vi "Load External Sources.vi"(8 "error in (no error)":errorcluster, 10 "JSON":string, 11 "BluelinesRedlines in":refnum<class "BluelinesRedlines.lvclass">) -> (0 "error out":errorcluster, 3 "BluelinesRedlines out":refnum<class "BluelinesRedlines.lvclass">)   [LabVIEW 2020, in "VolatusGUIElements.lvlib" / "BluelinesRedlines.lvclass"]
uses:
  BluelinesRedlines.lvclass
  BluelinesRedlines.lvclass/BluelinesRedlines.ctl
  <vilib>/JDP Science/JSONtext/Next JSON Value.vi
  <vilib>/JDP Science/JSONtext/String Subset.vi
  <vilib>/JDP Science/JSONtext/Parsing/Advance past next JSON Value (inlined COPY).vi
  <vilib>/JDP Science/JSONtext/Parsing/Advance past whitespace.vi
  <vilib>/JDP Science/JSONtext/Parsing/Advance past String.vi
  <vilib>/JDP Science/JSONtext/Parsing/Advance past Number.vi
  <vilib>/JDP Science/JSONtext/Parsing/Advance past Line Ending.vi
  <vilib>/JDP Science/JSONtext/Parsing/Parse Full Path or Item Name.vi
  <vilib>/JDP Science/JSONtext/Parsing/Advance past Array.vi
  <vilib>/JDP Science/JSONtext/Parsing/Advance past Object.vi
  <vilib>/JDP Science/JSONtext/support/Error Cluster From Code.vi
  <vilib>/JDP Science/JSONtext/Offset/Find Item Locations by Path.vi
  VolatusGUI/BluelinesRedlines Source/BluelinesRedlines Source.lvclass
  <vilib>/JDP Science/JSONtext/JSONtext.lvlib
  VolatusErrorUtilities/MultiErrors/MultiErrors.lvclass
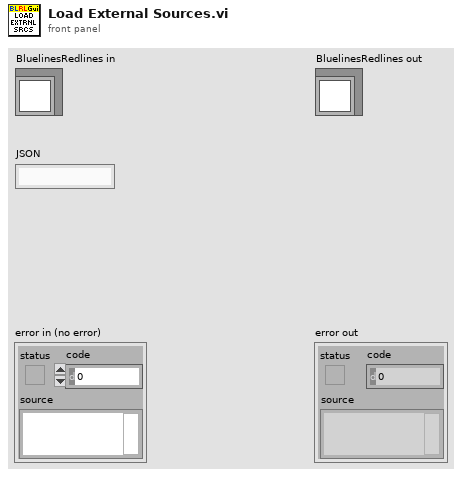
[diagram p1: front panel]
types:
  T1 = map{string, refnum<class "BluelinesRedlines Source.lvclass">}
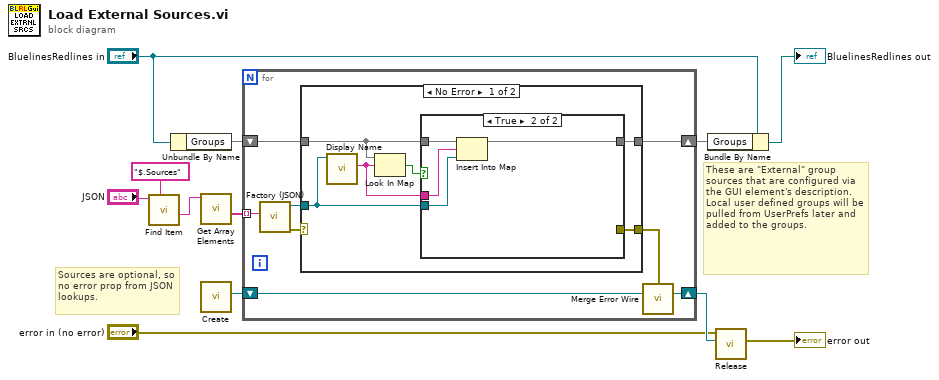
[diagram p0: block diagram]
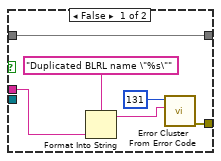
[diagram p2: hidden frame]
diagram:
  # "Sources are optional, so no error prop from JSON lookups."
  # "These are \"External\" group sources that are configured via the GUI element's description. Local user defined groups will be pulled from UserPrefs later and added to the groups."
  n1 = call <vilib>:"Find Item.vi"("$Path or Item Name"="$.Sources", "JSON"="JSON") -> ("<JSON>"=w10:string)  [unwired: 6 in, 3 out]
  n2 = Unbundle By Name("BluelinesRedlines in") -> ("Groups"=w1:T1)
  n3 = call <vilib>:"Get Array Elements.vi"("JSON"=w10) -> ("<JSON>"=w9:string[])  [unwired: 8 in, 2 out]
  n4 = call "Create.vi"() -> ("MultiErrors out"=w8:refnum<class "MultiErrors.lvclass">)  [unwired: 11 in]
  n5 = for {
    tunnel: w9 -> [w20] mode=indexing
    shift-right: [w17] -> w3
    shift-left: w1 -> [w18]
    shift-right: [w15] -> w7
    shift-left: w8 -> [w16]
    n6 = call "Factory (JSON).vi"("JSON"=w20) -> ("error out"=w14:errorcluster, "BLRL Source"=w19:refnum<class "BluelinesRedlines Source.lvclass">)  [unwired: 9 in]
    n7 = case shown="No Error" w14 {
      selector: w14 -> [_ w37]
      tunnel: w19 -> [w25 _]
      tunnel: w18 -> [w23 w38]
      tunnel: [w22 w38] -> w17
      tunnel: [w21 w37] -> w13
      frame No Error {
        n8 = call-dynamic "Display Name.vi"("BluelinesRedlines Source in"=w25) -> ("Display Name"=w24:string)  [unwired: 10 in]
        n9 = Look In Map(map=w23, key=w24) -> (key not found?=w26:bool)  [unwired: 1 in, 1 out]
        n10 = case shown="True" w26 {
          tunnel: w25 -> [_ w34]
          tunnel: w24 -> [w28 w35]
          tunnel: w23 -> [w32 w36]
          tunnel: [w32 w33] -> w22
          tunnel: [w30 _] -> w21
          frame False {
            n11 = Format Into String(format string="Duplicated BLRL name \"%s\"", w28) -> (resulting string=w29:string)  [unwired: 2 in, 1 out]
            n12 = call <vilib>:"Error Cluster From Error Code.vi"("error message (\"\")"=w29, "error code (0)"=131) -> ("error out"=w30:errorcluster)  [unwired: 7 in]
          }
          frame True {
            n13 = Insert Into Map(map in=w36, key=w35, value=w34) -> (map out=w33:T1)  [unwired: 2 out]
          }
        }
      }
      frame Error {
      }
    }
    n14 = call "Merge Error Wire.vi"("error in (no error)"=w13, "MultiErrors in"=w16) -> ("MultiErrors out"=w15:refnum<class "MultiErrors.lvclass">)  [unwired: 13 in]
  }
  n15 = Bundle By Name(cluster="BluelinesRedlines in", "Groups"=w3) -> (→"BluelinesRedlines out":refnum<class "BluelinesRedlines.lvclass">)
  n16 = call "Release.vi"("MultiErrors in"=w7, "Upstream Error (None)"="error in (no error)") -> ("error out"=→"error out":errorcluster)  [unwired: 9 in]
